vi "Msg.vi"(7 "jettl in":refnum<class "jettl.lvclass">, 11 "Last Ack Creator Queue Msg Strategy in":refnum<class "Last Ack Creator Queue Msg Strategy.lvclass">) -> (5 "jettl out":refnum<class "jettl.lvclass">)   [LabVIEW 2021, in "jettl.lvlib" / "Last Ack Creator Queue Msg Strategy.lvlib" / "Last Ack Creator Queue Msg Strategy.lvclass"]
uses:
  Last Ack Creator Queue Msg Strategy.lvclass
  jettl/jettl.lvclass
  jettl Msg Last Ack Creator Queue/jettl Msg Last Ack Creator Queue.lvclass
  Last Ack Creator Queue Msg Strategy.lvclass/Last Ack Creator Queue Msg Strategy.ctl
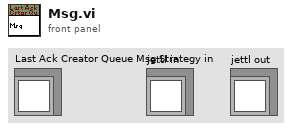
[diagram p1: front panel]
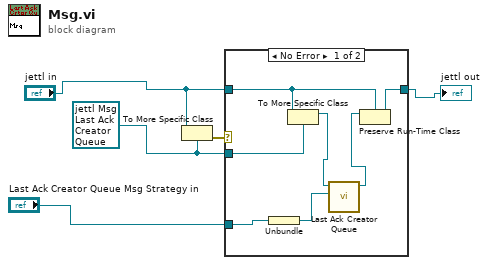
[diagram p0: block diagram]
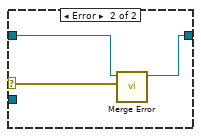
[diagram p2: hidden frame]
diagram:
  w1 = refnum<class "jettl Msg Last Ack Creator Queue.lvclass"> refnum ("jettl.lvlib:jettl Msg Last Ack Creator Queue.lvlib:jettl Msg Last Ack Creator Queue.lvclass")
  n1 = To More Specific Class(target class=w1, reference="jettl in") -> (error out=w5:errorcluster)  [unwired: 1 in, 1 out]
  n2 = case shown="No Error" w5 {
    selector: w5 -> [_ w15]
    tunnel: [w10 w13] -> w3
    tunnel: "jettl in" -> [w11 w14]
    tunnel: w1 -> [w12 _]
    tunnel: "Last Ack Creator Queue Msg Strategy in" -> [w9 _]
    frame No Error {
      n3 = Unbundle(w9) -> (w6:refnum<class "Queue.lvclass">)
      n4 = To More Specific Class(target class=w12, reference=w11) -> (specific class reference=w8:refnum<class "jettl Msg Last Ack Creator Queue.lvclass">)  [unwired: 1 in, 1 out]
      n5 = call-dynamic "Last Ack Creator Queue.vi"("Queue"=w6, "jettl Msg Last Ack Creator Queue in"=w8) -> ("jettl Msg Last Ack Creator Queue out"=w7:refnum<class "jettl Msg Last Ack Creator Queue.lvclass">)  [unwired: 9 in]
      n6 = Preserve Run-Time Class(object in=w7, 2:w11) -> (object out=w10:refnum<class "jettl.lvclass">)  [unwired: 1 in, 1 out]
    }
    frame Error {
      n7 = call-dynamic "Merge Error.vi"("Error"=w15, "jettl Msg Merge Error in"=w14) -> ("jettl Msg Merge Error out"=w13:refnum<class "jettl.lvclass">)  [unwired: 9 in]
    }
  }
  "jettl out" <- w3
